vi "Init UI.vi"(8 "error in (no error)":errorcluster, 11 "Configuration Window in":refnum<class "Configuration Window.lvclass">) -> (0 "error out":errorcluster, 3 "Configuration Window out":refnum<class "Configuration Window.lvclass">)   [LabVIEW 2018, in "Configuration Window.lvlib" / "Configuration Window.lvclass"]
uses:
  Configuration Window.lvclass
  Configuration Window.lvclass/Configuration Window.ctl
  <userlib>/_OpenG.lib/file/file.llb/Strip Path Extension - 1D Array of Strings__ogtk.vi
  Framework/Framework/Framework.lvclass
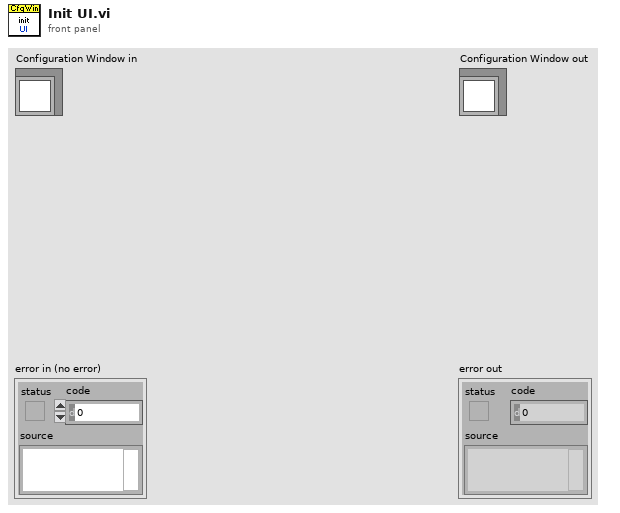
[diagram p1: front panel]
types:
  T1 = cluster{"Name":refnum<vi>, "Size":refnum<vi>, "Color":refnum<vi>, "Enable":refnum<vi>}
  T2 = cluster{"Name":refnum<vi>, "Fill Color":refnum<vi>, "Border Color":refnum<vi>, "Enable":refnum<vi>}
  T3 = cluster{"Fill Color":u32, "Border Color":u32, "Show?":bool}
  T4 = cluster{"Reset to Steam Path":refnum<vi>, "_res_data":refnum<vi>, "_res_pngs":refnum<vi>, "mp3":refnum<vi>}
  T5 = typedef "Main Panel.lvlib/Main Panel.lvclass/Const Path Setting.ctl" = cluster{"Data Folder Path":path, "PNG Folder Path":path, "mp3 Folder Path":path}
  T6 = typedef "Framework.lvlib/Framework.lvclass/Const Lang Setting.ctl" = cluster{"Main Panel":T7, "Configuration Window":T20}
  T7 = typedef "Framework.lvlib/Framework.lvclass/Const Lang MainWnd.ctl" = cluster{"Title":T8, "Frame Basic":T10, "Frame Skill":T11, "bp":T12, "w":T13, "b":T14, "i":T15, "o":T16, "c":T17, "Other":T18, "Menu":T19}
  T8 = typedef "Framework.lvlib/Framework.lvclass/Const Lang MainWnd Frame Title.ctl" = cluster{"Frame Num":T9, "Name":T9}
  T9 = typedef "Framework.lvlib/Framework.lvclass/Const Lang Property.ctl" = cluster{"Name":string, "Tip":string, "Description":string}
  T10 = typedef "Framework.lvlib/Framework.lvclass/Const Lang MainWnd Frame Basic.ctl" = cluster{"pic":T9, "state":T9, "wait":T9, "next":T9, "dvx":T9, "dvy":T9, "dvz":T9, "centerx":T9, "centery":T9, "sound":T9}
  T11 = typedef "Framework.lvlib/Framework.lvclass/Const Lang MainWnd Frame Skill.ctl" = cluster{"mp":T9, "hit_a":T9, "hit_d":T9, "hit_j":T9, "hit_Fa":T9, "hit_Ua":T9, "hit_Da":T9, "hit_Fj":T9, "hit_Uj":T9, "hit_Dj":T9, "hit_ja":T9}
  T12 = typedef "Framework.lvlib/Framework.lvclass/Const Lang MainWnd Frame bp.ctl" = cluster{"x":T9, "y":T9}
  T13 = typedef "Framework.lvlib/Framework.lvclass/Const Lang MainWnd Frame w.ctl" = cluster{"kind":T9, "x":T9, "y":T9, "weaponact":T9, "cover":T9, "dvx":T9, "dvy":T9, "dvz":T9, "attacking":T9}
  T14 = typedef "Framework.lvlib/Framework.lvclass/Const Lang MainWnd Frame b.ctl" = cluster{"kind":T9, "x":T9, "y":T9, "w":T9, "h":T9, "index":T9}
  T15 = typedef "Framework.lvlib/Framework.lvclass/Const Lang MainWnd Frame i.ctl" = cluster{"kind":T9, "x":T9, "y":T9, "w":T9, "h":T9, "zwidth":T9, "dvx":T9, "dvy":T9, "dvz":T9, "fall":T9, "arest":T9, "vrest":T9, "bdefend":T9, "injury":T9, "effect":T9, "catchingact 1":T9, "catchingact 2":T9, "caughtact 1":T9, "caughtact 2":T9, "index":T9}
  T16 = typedef "Framework.lvlib/Framework.lvclass/Const Lang MainWnd Frame o.ctl" = cluster{"kind":T9, "x":T9, "y":T9, "action":T9, "dvx":T9, "dvy":T9, "dvz":T9, "oid":T9, "facing":T9}
  T17 = typedef "Framework.lvlib/Framework.lvclass/Const Lang MainWnd Frame c.ctl" = cluster{"kind":T9, "x":T9, "y":T9, "injury":T9, "cover":T9, "vaction":T9, "aaction":T9, "taction":T9, "hurtable":T9, "decrease":T9, "fronthurtact":T9, "backhurtact":T9, "throwvx":T9, "throwvy":T9, "throwvz":T9, "throwinjury":T9, "dircontrol":T9}
  T18 = typedef "Framework.lvlib/Framework.lvclass/Const Lang MainWnd Other.ctl" = cluster{"File Path":T9, "GoTo":T9, "Apply Change":T9, "To Next Frame":T9, "Sound Play":T9}
  T19 = typedef "Framework.lvlib/Framework.lvclass/Const Lang MainWnd Menu.ctl" = cluster{"File":T9, "Open File":T9, "Save File":T9, "Exit":T9, "Settings":T9, "Preferences":T9, "Tool":T9, "Pic Json Generator":T9, "Help":T9, "Show Context Help":T9}
  T20 = typedef "Framework.lvlib/Framework.lvclass/Const Lang CfgWnd.ctl" = cluster{"Tab":T21, "Main":T22, "Path":T23, "Image":T24}
  T21 = typedef "Framework.lvlib/Framework.lvclass/Const Lang CfgWnd Tab.ctl" = cluster{"Main Page":T9, "Image Page":T9}
  T22 = typedef "Framework.lvlib/Framework.lvclass/Const Lang CfgWnd Main.ctl" = cluster{"Language":T9, "Save":T9, "Cancel":T9}
  T23 = typedef "Framework.lvlib/Framework.lvclass/Const Lang CfgWnd Path.ctl" = cluster{"Reset":T9, "Path Data":T9, "Path Png":T9, "Path Mp3":T9}
  T24 = typedef "Framework.lvlib/Framework.lvclass/Const Lang CfgWnd Image.ctl" = cluster{"Center Point":cluster{"Name":T9, "Size":T9, "Color":T9, "Enable":T9}, "bp Point":cluster{"Name":T9, "Size":T9, "Color":T9, "Enable":T9}, "w Point":cluster{"Name":T9, "Size":T9, "Color":T9, "Enable":T9}, "b Box":cluster{"Name":T9, "Fill Color":T9, "Border Color":T9, "Enable":T9}, "i Box":cluster{"Name":T9, "Fill Color":T9, "Border Color":T9, "Enable":T9}, "o Point":cluster{"Name":T9, "Size":T9, "Color":T9, "Enable":T9}, "c Point":cluster{"Name":T9, "Size":T9, "Color":T9, "Enable":T9}}
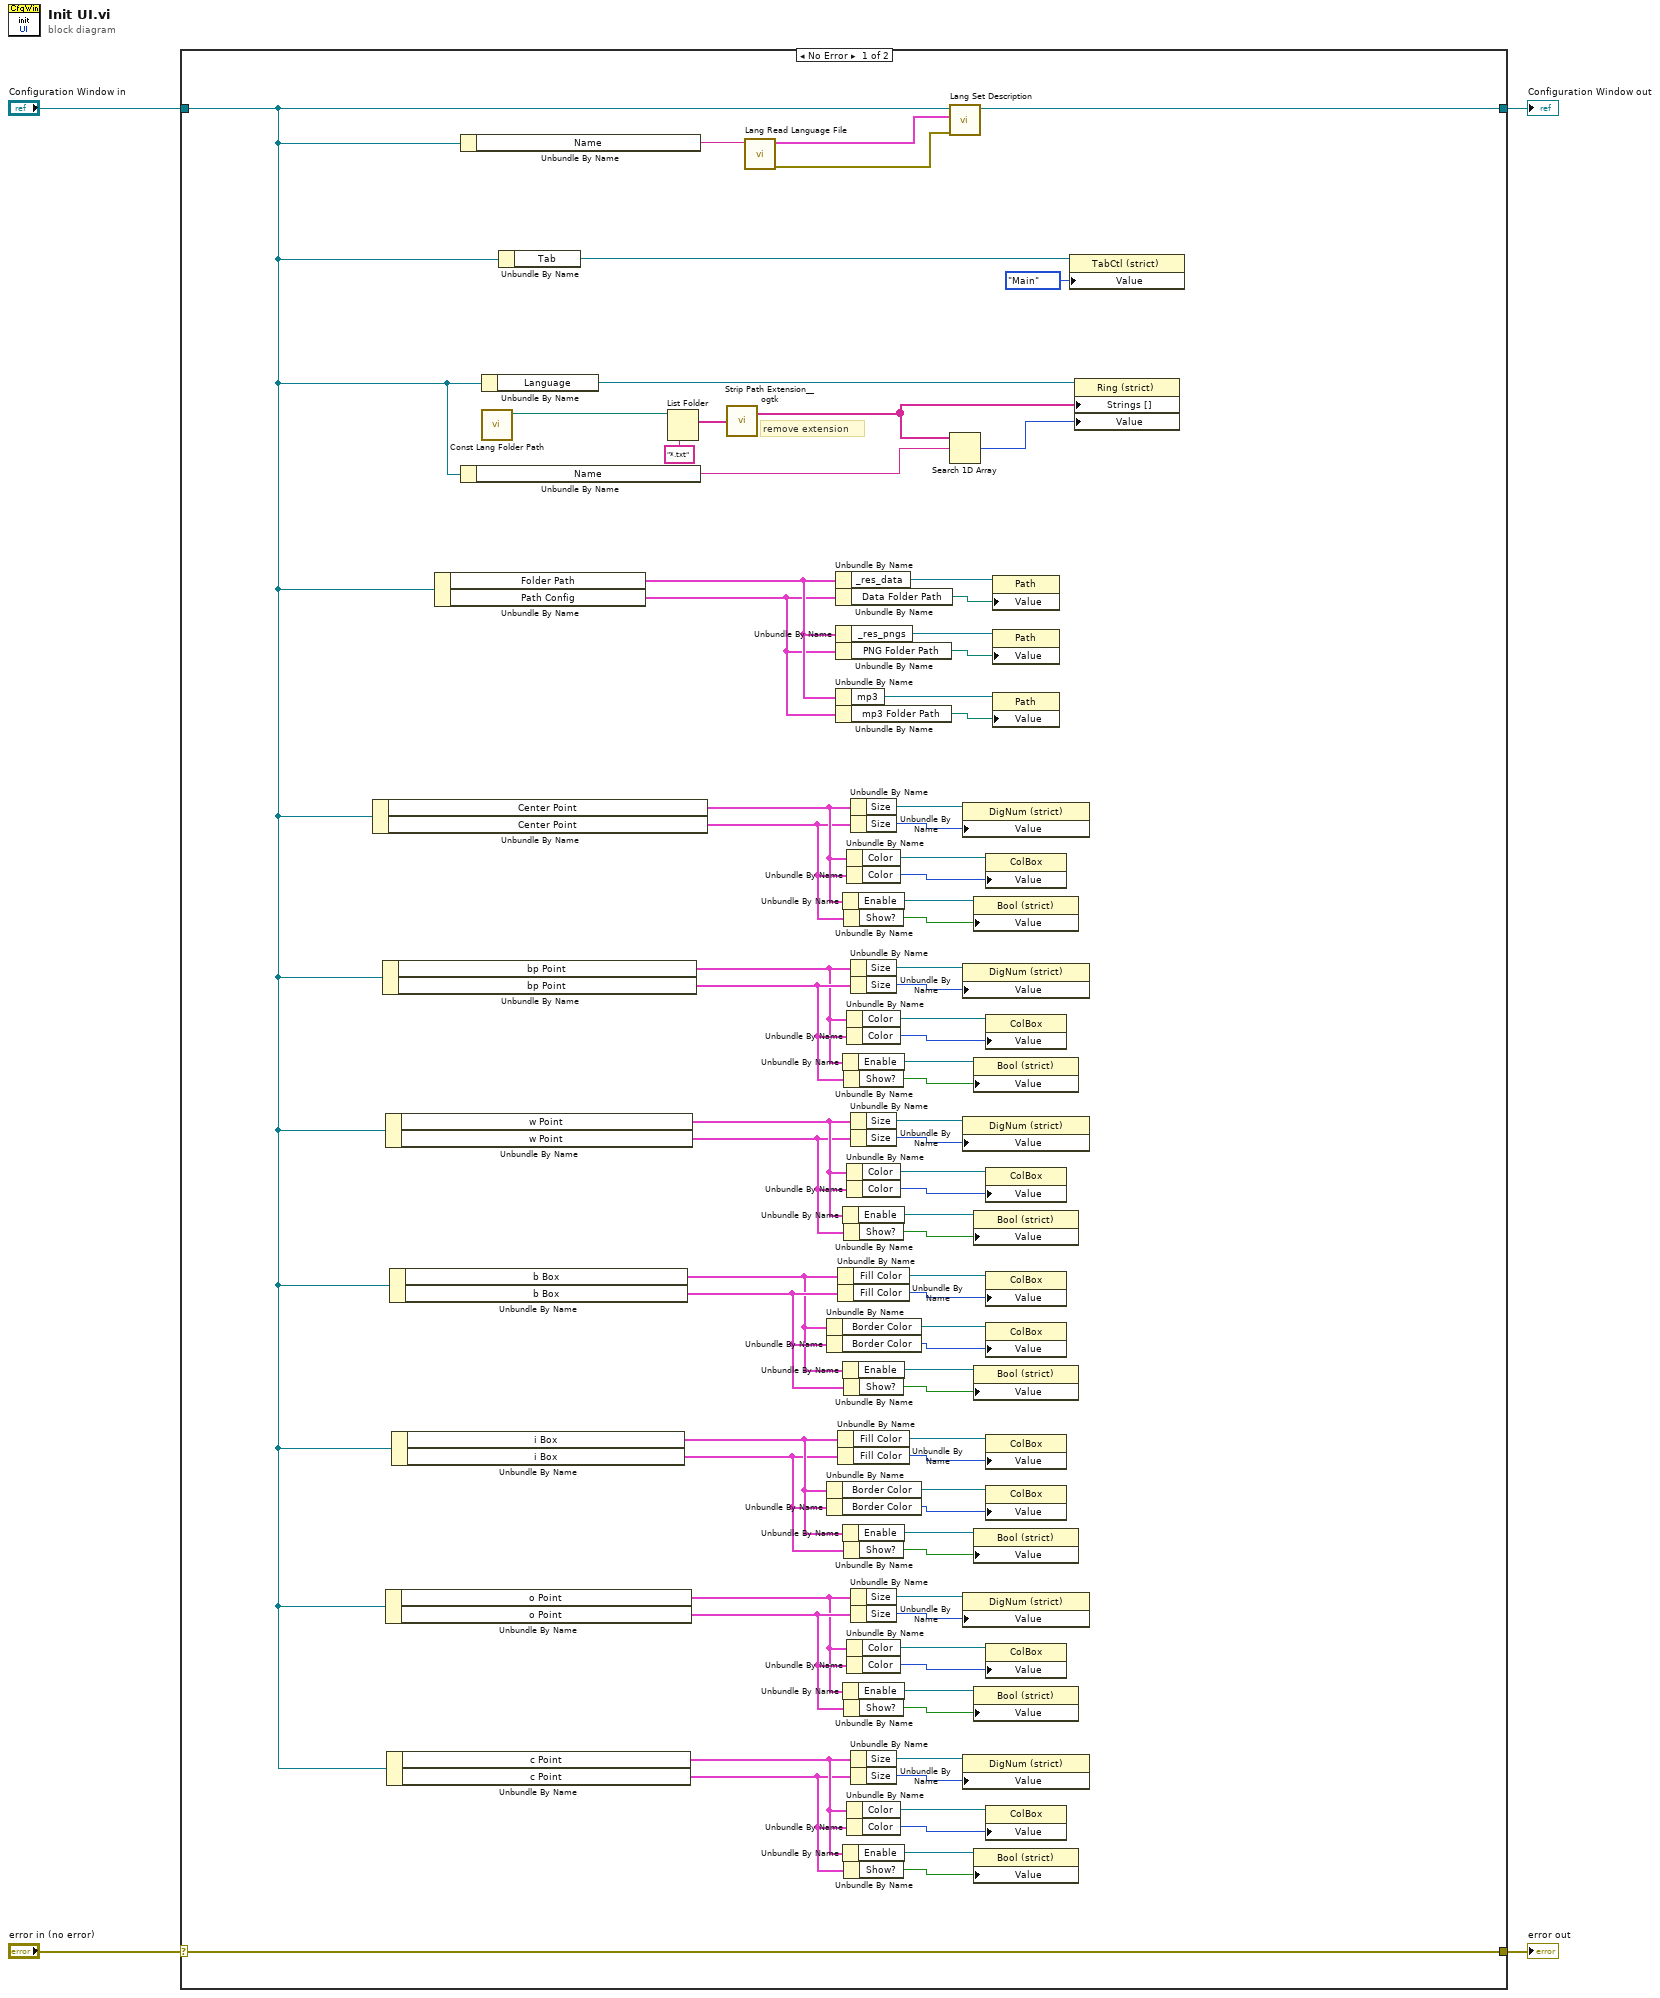
[diagram p0: block diagram]
diagram:
  n1 = case shown="No Error" "error in (no error)" {
    selector: "error in (no error)" -> [w83 w85]
    tunnel: [w83 w85] -> w3
    tunnel: [w14 w84] -> w1
    tunnel: "Configuration Window in" -> [w11 w84]
    frame No Error {
      # "remove extension"
      n2 = Unbundle By Name(w11) -> ("Center Point"=w72:T1, "Center Point"=w71:cluster{"Size":i32, "Color":u32, "Show?":bool})
      n3 = Unbundle By Name(w11) -> ("bp Point"=w69:T1, "bp Point"=w70:cluster{"Size":i32, "Color":u32, "Show?":bool})
      n4 = Unbundle By Name(w11) -> ("w Point"=w56:T1, "w Point"=w55:cluster{"Size":i32, "Color":u32, "Show?":bool})
      n5 = Unbundle By Name(w11) -> ("o Point"=w37:T1, "o Point"=w38:cluster{"Size":i32, "Color":u32, "Show?":bool})
      n6 = Unbundle By Name(w11) -> ("c Point"=w24:T1, "c Point"=w23:cluster{"Size":i32, "Color":u32, "Show?":bool})
      n7 = Unbundle By Name(w11) -> ("b Box"=w53:T2, "b Box"=w54:T3)
      n8 = Unbundle By Name(w11) -> ("i Box"=w40:T2, "i Box"=w39:T3)
      n9 = Unbundle By Name(w11) -> ("Folder Path"=w6:T4, "Path Config"=w5:T5)
      n10 = Unbundle By Name(w11) -> ("Name"=w15:string)
      n11 = Unbundle By Name(w11) -> ("Name"=w16:string)
      n12 = Unbundle By Name(w11) -> ("Language"=w22:refnum<vi>)
      n13 = call "Const Lang Folder Path.vi"() -> ("Language Folder Path"=w21:path)  [unwired: 11 in]
      n14 = Unbundle By Name(w11) -> ("Tab"=w10:refnum<vi>)
      n15 = List Folder(path=w21, pattern="*.txt") -> (filenames=w19:string[])  [unwired: 2 in, 3 out]
      n16 = call-poly <userlib>:"Strip Path Extension__ogtk.vi"("paths"=w19) -> ("roots"=w17:string[])  [unwired: 1 out]
      n17 = call "Lang Read Language File.vi"("Language Name"=w15) -> ("error out"=w12:errorcluster, "UI Descriptions"=w13:T6)  [unwired: 8 in, 1 out]
      n18 = Unbundle By Name(w53) -> ("Border Color"=w50:refnum<vi>)
      n19 = Unbundle By Name(w54) -> ("Border Color"=w49:u32)
      n20 = Unbundle By Name(w40) -> ("Border Color"=w43:refnum<vi>)
      n21 = Unbundle By Name(w39) -> ("Border Color"=w44:u32)
      n22 = Unbundle By Name(w6) -> ("_res_data"=w82:refnum<vi>)
      n23 = Unbundle By Name(w5) -> ("Data Folder Path"=w81:path)
      n24 = Unbundle By Name(w6) -> ("_res_pngs"=w79:refnum<vi>)
      n25 = Unbundle By Name(w5) -> ("PNG Folder Path"=w80:path)
      n26 = Unbundle By Name(w6) -> ("mp3"=w8:refnum<vi>)
      n27 = Unbundle By Name(w5) -> ("mp3 Folder Path"=w7:path)
      n28 = Unbundle By Name(w53) -> ("Fill Color"=w47:refnum<vi>)
      n29 = Unbundle By Name(w54) -> ("Fill Color"=w48:u32)
      n30 = Unbundle By Name(w40) -> ("Fill Color"=w46:refnum<vi>)
      n31 = Unbundle By Name(w39) -> ("Fill Color"=w45:u32)
      n32 = Unbundle By Name(w72) -> ("Enable"=w74:refnum<vi>)
      n33 = Unbundle By Name(w69) -> ("Enable"=w67:refnum<vi>)
      n34 = Unbundle By Name(w56) -> ("Enable"=w58:refnum<vi>)
      n35 = Unbundle By Name(w53) -> ("Enable"=w51:refnum<vi>)
      n36 = Unbundle By Name(w40) -> ("Enable"=w42:refnum<vi>)
      n37 = Unbundle By Name(w37) -> ("Enable"=w35:refnum<vi>)
      n38 = Unbundle By Name(w24) -> ("Enable"=w26:refnum<vi>)
      n39 = Unbundle By Name(w71) -> ("Show?"=w73:bool)
      n40 = Unbundle By Name(w70) -> ("Show?"=w68:bool)
      n41 = Unbundle By Name(w55) -> ("Show?"=w57:bool)
      n42 = Unbundle By Name(w54) -> ("Show?"=w52:bool)
      n43 = Unbundle By Name(w39) -> ("Show?"=w41:bool)
      n44 = Unbundle By Name(w38) -> ("Show?"=w36:bool)
      n45 = Unbundle By Name(w23) -> ("Show?"=w25:bool)
      n46 = Unbundle By Name(w72) -> ("Color"=w75:refnum<vi>)
      n47 = Unbundle By Name(w71) -> ("Color"=w76:u32)
      n48 = Unbundle By Name(w69) -> ("Color"=w66:refnum<vi>)
      n49 = Unbundle By Name(w70) -> ("Color"=w65:u32)
      n50 = Unbundle By Name(w56) -> ("Color"=w59:refnum<vi>)
      n51 = Unbundle By Name(w55) -> ("Color"=w60:u32)
      n52 = Unbundle By Name(w37) -> ("Color"=w34:refnum<vi>)
      n53 = Unbundle By Name(w38) -> ("Color"=w33:u32)
      n54 = Unbundle By Name(w24) -> ("Color"=w27:refnum<vi>)
      n55 = Unbundle By Name(w23) -> ("Color"=w28:u32)
      n56 = Unbundle By Name(w72) -> ("Size"=w78:refnum<vi>)
      n57 = Unbundle By Name(w71) -> ("Size"=w77:i32)
      n58 = Unbundle By Name(w69) -> ("Size"=w63:refnum<vi>)
      n59 = Unbundle By Name(w70) -> ("Size"=w64:i32)
      n60 = Unbundle By Name(w56) -> ("Size"=w62:refnum<vi>)
      n61 = Unbundle By Name(w55) -> ("Size"=w61:i32)
      n62 = Unbundle By Name(w37) -> ("Size"=w31:refnum<vi>)
      n63 = Unbundle By Name(w38) -> ("Size"=w32:i32)
      n64 = Unbundle By Name(w24) -> ("Size"=w30:refnum<vi>)
      n65 = Unbundle By Name(w23) -> ("Size"=w29:i32)
      n66 = call "Lang Set Description.vi"("error in (no error)"=w12, "UI Descriptions"=w13, "Configuration Window in"=w11) -> ("Configuration Window out"=w14:refnum<class "Configuration Window.lvclass">)  [unwired: 7 in, 1 out]
      n67 = Search 1D Array(1D array=w17, element=w16) -> (index of element=w18:i32)  [unwired: 1 in]
      n68 = property class="DigNum (strict)"(reference=w78, "Value"=w77) -> ()  [unwired: 1 in, 2 out]
      n69 = property class="DigNum (strict)"(reference=w63, "Value"=w64) -> ()  [unwired: 1 in, 2 out]
      n70 = property class="DigNum (strict)"(reference=w62, "Value"=w61) -> ()  [unwired: 1 in, 2 out]
      n71 = property class="DigNum (strict)"(reference=w31, "Value"=w32) -> ()  [unwired: 1 in, 2 out]
      n72 = property class="DigNum (strict)"(reference=w30, "Value"=w29) -> ()  [unwired: 1 in, 2 out]
      n73 = property class="Bool (strict)"(reference=w74, "Value"=w73) -> ()  [unwired: 1 in, 2 out]
      n74 = property class="Bool (strict)"(reference=w67, "Value"=w68) -> ()  [unwired: 1 in, 2 out]
      n75 = property class="Bool (strict)"(reference=w58, "Value"=w57) -> ()  [unwired: 1 in, 2 out]
      n76 = property class="Bool (strict)"(reference=w51, "Value"=w52) -> ()  [unwired: 1 in, 2 out]
      n77 = property class="Bool (strict)"(reference=w42, "Value"=w41) -> ()  [unwired: 1 in, 2 out]
      n78 = property class="Bool (strict)"(reference=w35, "Value"=w36) -> ()  [unwired: 1 in, 2 out]
      n79 = property class="Bool (strict)"(reference=w26, "Value"=w25) -> ()  [unwired: 1 in, 2 out]
      n80 = property class="ColBox"(reference=w75, "Value"=w76) -> ()  [unwired: 1 in, 2 out]
      n81 = property class="ColBox"(reference=w66, "Value"=w65) -> ()  [unwired: 1 in, 2 out]
      n82 = property class="ColBox"(reference=w59, "Value"=w60) -> ()  [unwired: 1 in, 2 out]
      n83 = property class="ColBox"(reference=w47, "Value"=w48) -> ()  [unwired: 1 in, 2 out]
      n84 = property class="ColBox"(reference=w50, "Value"=w49) -> ()  [unwired: 1 in, 2 out]
      n85 = property class="ColBox"(reference=w46, "Value"=w45) -> ()  [unwired: 1 in, 2 out]
      n86 = property class="ColBox"(reference=w43, "Value"=w44) -> ()  [unwired: 1 in, 2 out]
      n87 = property class="ColBox"(reference=w34, "Value"=w33) -> ()  [unwired: 1 in, 2 out]
      n88 = property class="ColBox"(reference=w27, "Value"=w28) -> ()  [unwired: 1 in, 2 out]
      n89 = property class="Path"(reference=w82, "Value"=w81) -> ()  [unwired: 1 in, 2 out]
      n90 = property class="Path"(reference=w79, "Value"=w80) -> ()  [unwired: 1 in, 2 out]
      n91 = property class="Path"(reference=w8, "Value"=w7) -> ()  [unwired: 1 in, 2 out]
      n92 = property class="TabCtl (strict)"(reference=w10, "Value"=enum32{"Main", "Image"}."Main") -> ()  [unwired: 1 in, 2 out]
      n93 = property class="Ring (strict)"(reference=w22, "Strings []"=w17, "Value"=w18) -> ()  [unwired: 1 in, 2 out]
    }
    frame Error {
    }
  }
  "error out" <- w3
  "Configuration Window out" <- w1
